vi "string parse mathematica assosiated array.vi"(7 "derivative":T2=enum."parse string", 10 "Map IN":map{T1, dbl}(c390), 11 "String in":string="74 -> <|\"m1\" -> 0.144686311901723`, \"m2\" -> 0.01872411095198769`, \n  \"m3\" -> 0.00012732395447351627`, \"T\" -> 0.249000, \n  \"\\[Zeta]\" -> 0.077915, \"\\[Tau]1\" -> 0.054530, \"\\[Tau]S\" -> 0.034022,\n   \"\\[Tau]N\" -> 0.048248, \"\\[Tau]C\" -> 0.002031, \n  \"\\[Kappa]0\" -> 0.000000001550, \"mm1\" -> 0.016334, \"mm2\" -> 0.128767,\n   \"mm3\" -> 0.000140|>,\n\n\n") -> (2 "Map OUT":map{T1, dbl}(c390), 3 "String OUT":string)   [LabVIEW 2020]
uses:
  3-lorentzian-parameters.ctl
  mathematica string map action.ctl
  3-lorentzian-heat-response action.ctl
  <vilib>/regexp/Match Regular Expression.xnode
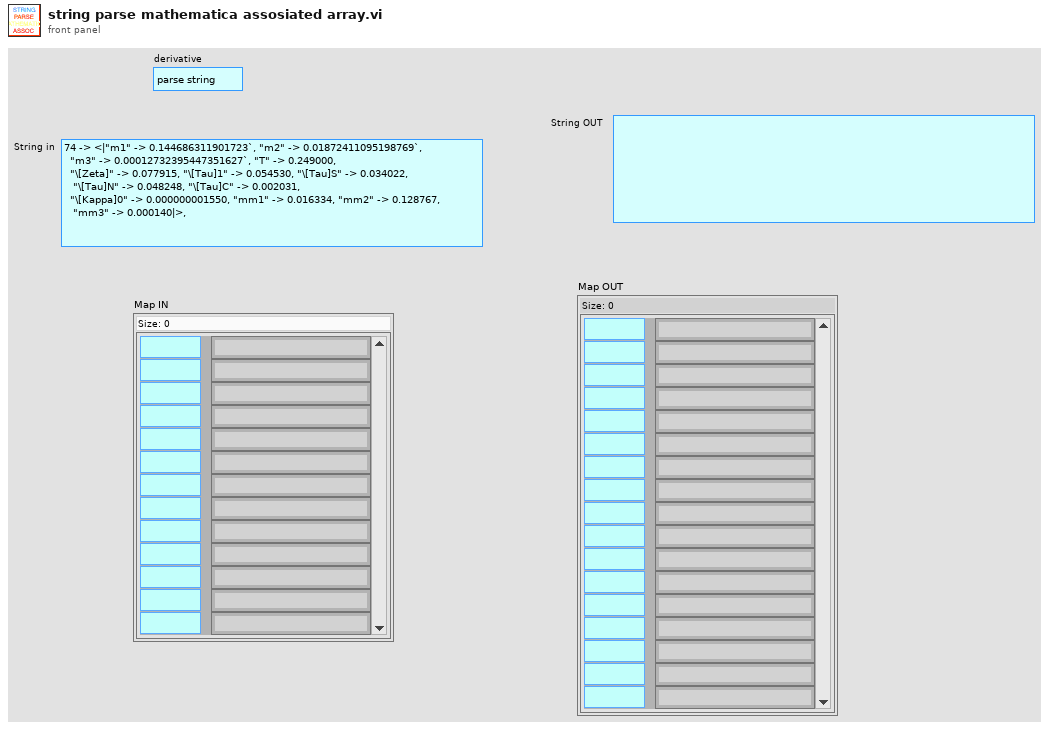
[diagram p1: front panel]
types:
  T1 = typedef "3-lorentzian-parameters.ctl" = enum16{"ζ", "τ1", "τS", "τN", "τC", "κ0", "m1", "m2", "m3", "T (K)", "B (T)", "θ (deg)"}
  T2 = typedef "mathematica string map action.ctl" = enum16{"create string", "calc m1m2m3", "parse string"}
  T3 = typedef "3-lorentzian-heat-response action.ctl" = enum16{"calc R", "create string", "calc m1m2m3", "dζ", "dT1", "dτS", "dτN", "dτC", "d-all", "dκ0", "T(K)", "m1", "m2", "m3", "parse string", "θ (deg)", "B (T)", "onlygrads"}
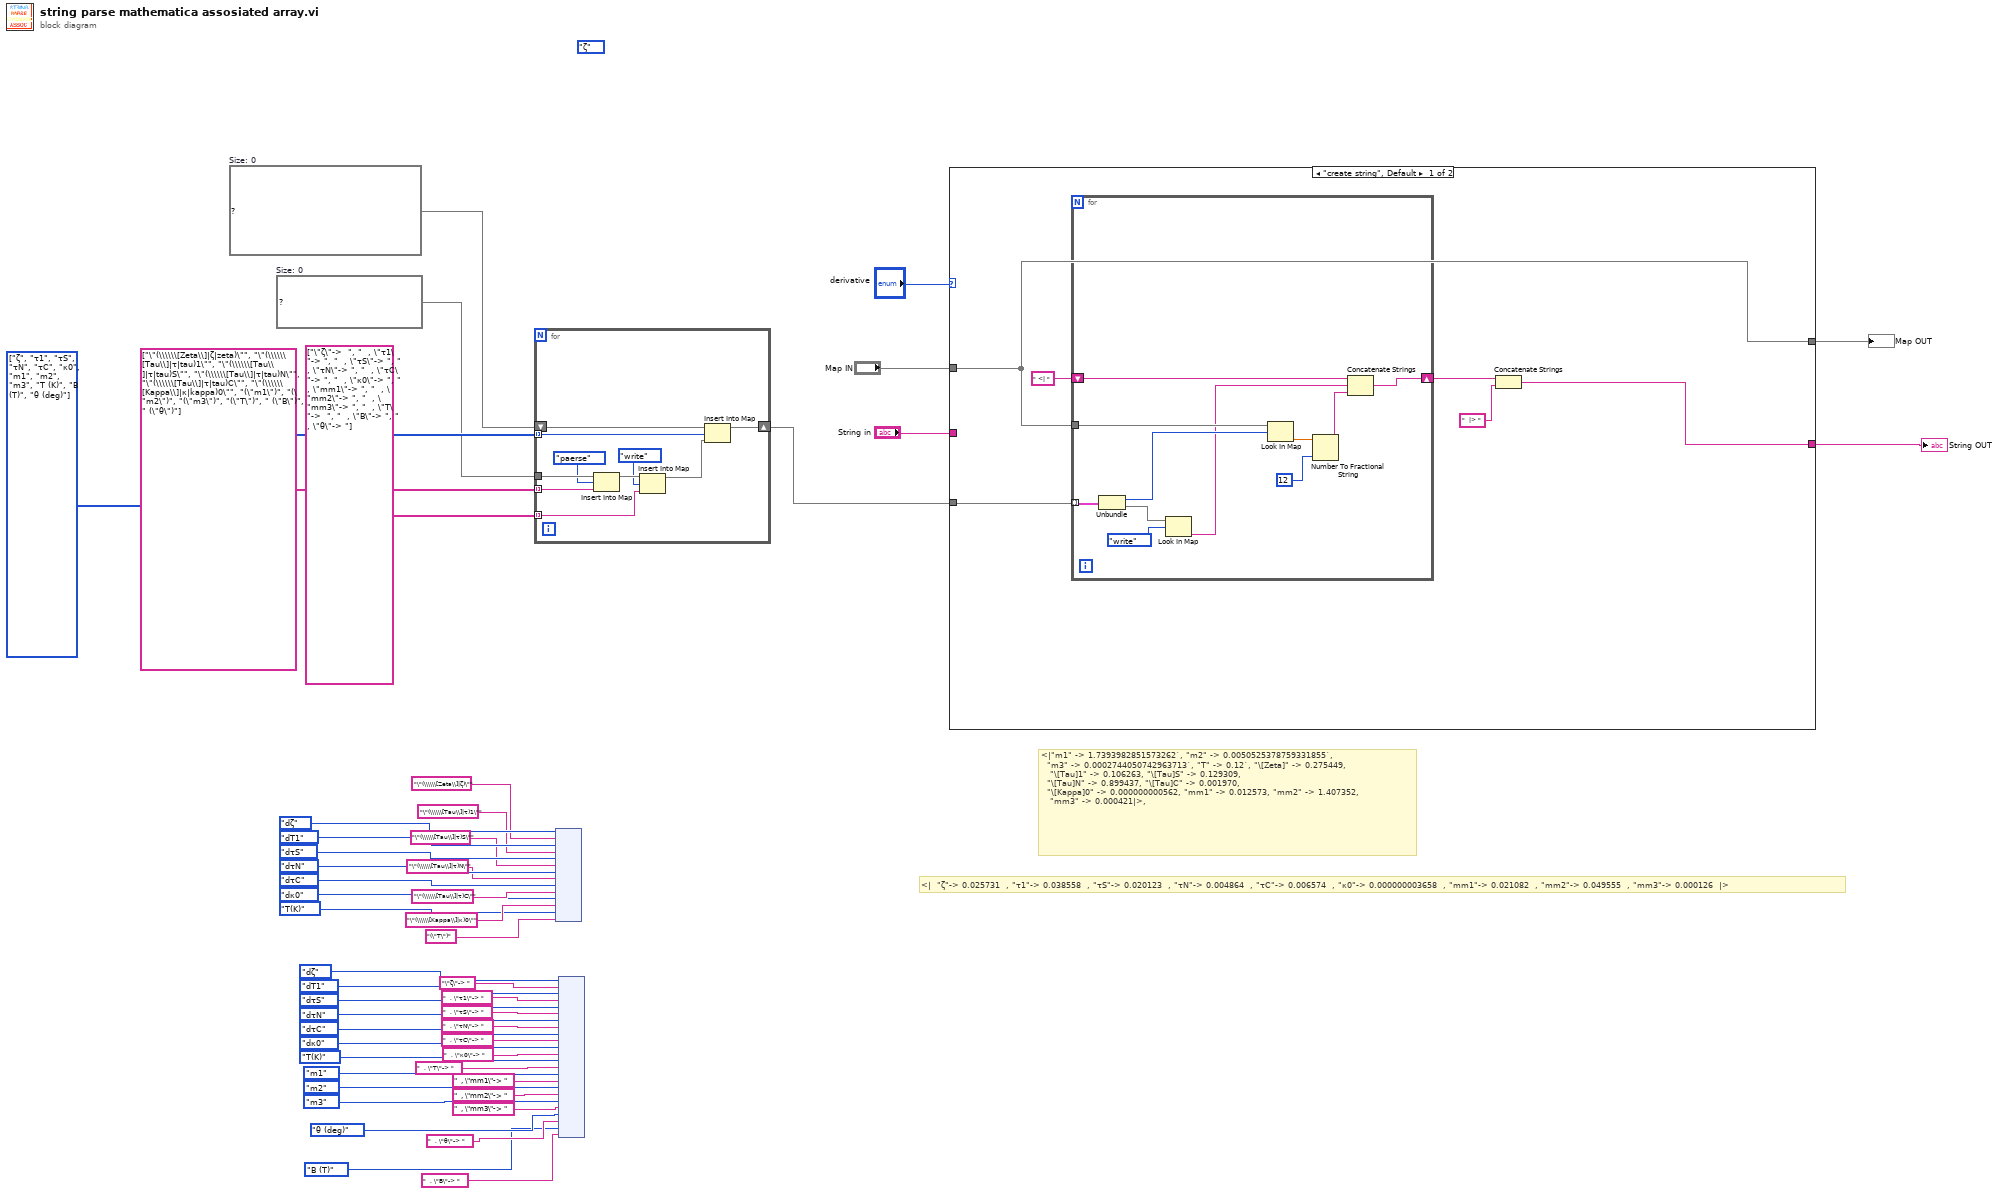
[diagram p0: block diagram]
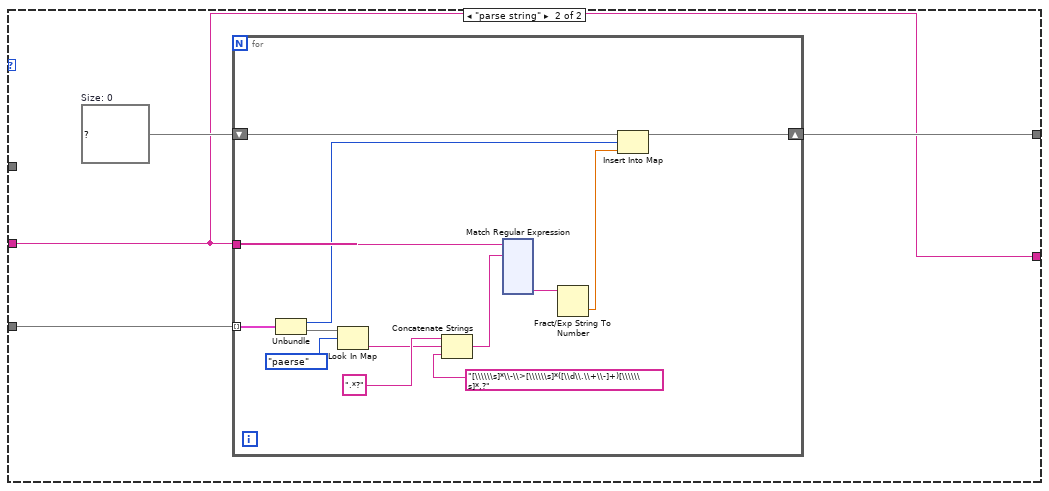
[diagram p2: hidden frame]
diagram:
  (unwired) 3-lorentzian-parameters."ζ" ("what")
  w5 = map{enum16{"paerse", "write"}, string} {}  # Size: 0
  w6 = map{T1, map{enum16{"paerse", "write"}, string}} {}  # Size: 0
  w7 = T1[] [enum."ζ", enum."τ1", enum."τS", enum."τN", enum."τC", enum."κ0", enum."m1", enum."m2", enum."m3", enum."T (K)", enum."B (T)", enum."θ (deg)"] items=["ζ", "τ1", "τS", "τN", "τC", "κ0", "m1", "m2", "m3", "T (K)", "B (T)", "θ (deg)"]
  # "<|\"m1\" -> 1.7393982851573262`, \"m2\" -> 0.0050525378759331855`, \n  \"m3\" -> 0.0002744050742963713`, \"T\" -> 0.12`, \"\\[Zeta]\" -> 0.275449,\n   \"\\[Tau]1\" -> 0.106263, \"\\[Tau]S\" -> 0.129309, \n  \"\\[Tau]N\" -> 0.899437, \"\\[Tau]C\" -> 0.001970, \n  \"\\[Kappa]0\" -> 0.000000000562, \"mm1\" -> 0.012573, \"mm2\" -> 1.407352,\n   \"mm3\" -> 0.000421|>,"
  # "<|  \"ζ\"-> 0.025731  , \"τ1\"-> 0.038558  , \"τS\"-> 0.020123  , \"τN\"-> 0.004864  , \"τC\"-> 0.006574  , \"κ0\"-> 0.000000003658  , \"mm1\"-> 0.021082  , \"mm2\"-> 0.049555  , \"mm3\"-> 0.000126  |>"
  n1 = for {
    tunnel: w7 -> [w57] mode=indexing
    shift-right: [w58] -> w2
    shift-left: w6 -> [w59]
    tunnel: w5 -> [w56]
    tunnel: string[] ["\"(\\\\\\[Zeta\\]|ζ|zeta)\"", "\"(\\\\\\[Tau\\]|τ|tau)1\"", "\"(\\\\\\[Tau\\]|τ|tau)S\"", "\"(\\\\\\[Tau\\]|τ|tau)N\"", "\"(\\\\\\[Tau\\]|τ|tau)C\"", "\"(\\\\\\[Kappa\\]|κ|kappa)0\"", "(\"m1\")", "(\"m2\")", "(\"m3\")", "(\"T\")", " (\"B\")", " (\"θ\")"] -> [w51] mode=indexing
    tunnel: string[] ["\"ζ\"->  ", "  , \"τ1\"-> ", "  , \"τS\"-> ", "  , \"τN\"-> ", "  , \"τC\"-> ", "  , \"κ0\"-> ", "  , \"mm1\"-> ", "  , \"mm2\"-> ", "  , \"mm3\"-> ", "  , \"T\"->  ", "  , \"B\"-> ", "  , \"θ\"-> "] -> [w50] mode=indexing
    n2 = Insert Into Map(map in=w56, key=enum16{"paerse", "write"}."paerse", value=w51) -> (map out=w55:map{enum16{"paerse", "write"}, string})  [unwired: 2 out]
    n3 = Insert Into Map(map in=w55, key=enum16{"paerse", "write"}."write", value=w50) -> (map out=w54:map{enum16{"paerse", "write"}, string})  [unwired: 2 out]
    n4 = Insert Into Map(map in=w59, key=w57, value=w54) -> (map out=w58:map{T1, map{enum16{"paerse", "write"}, string}})  [unwired: 2 out]
  }
  n5 = node(3-lorentzian-heat-response_action."dζ" ("derivative"), "\"(\\\\\\[Zeta\\]|ζ)\"" ("format string"), 3-lorentzian-heat-response_action."dT1" ("derivative"), "\"(\\\\\\[Tau\\]|τ)1\"" ("format string"), 3-lorentzian-heat-response_action."dτS" ("derivative"), "\"(\\\\\\[Tau\\]|τ)S\"" ("format string"), 3-lorentzian-heat-response_action."dτN" ("derivative"), "\"(\\\\\\[Tau\\]|τ)N\"" ("format string"), 3-lorentzian-heat-response_action."dτC" ("derivative"), "\"(\\\\\\[Tau\\]|τ)C\"" ("format string"), 3-lorentzian-heat-response_action."dκ0" ("derivative"), "\"(\\\\\\[Kappa\\]|κ)0\"" ("format string"), 3-lorentzian-heat-response_action."T(K)" ("derivative"), "(\"T\")" ("format string")) -> ()  [unwired: 1 out]
  n6 = node(3-lorentzian-heat-response_action."dζ" ("derivative"), "\"ζ\"-> ", 3-lorentzian-heat-response_action."dT1" ("derivative"), "  , \"τ1\"-> ", 3-lorentzian-heat-response_action."dτS" ("derivative"), "  , \"τS\"-> ", 3-lorentzian-heat-response_action."dτN" ("derivative"), "  , \"τN\"-> ", 3-lorentzian-heat-response_action."dτC" ("derivative"), "  , \"τC\"-> ", 3-lorentzian-heat-response_action."dκ0" ("derivative"), "  , \"κ0\"-> ", 3-lorentzian-heat-response_action."T(K)" ("derivative"), "  , \"T\"-> ", 3-lorentzian-heat-response_action."m1" ("derivative"), "  , \"mm1\"-> ", 3-lorentzian-heat-response_action."m2" ("derivative"), "  , \"mm2\"-> ", 3-lorentzian-heat-response_action."m3" ("derivative"), "  , \"mm3\"-> ", 3-lorentzian-heat-response_action."θ (deg)" ("derivative"), "  , \"θ\"-> ", 3-lorentzian-heat-response_action."B (T)" ("derivative"), "  , \"B\"-> ") -> ()  [unwired: 1 out]
  n7 = case shown="\"create string\", Default" "derivative" {
    tunnel: "String in" -> [_ w78]
    tunnel: [w61 w79] -> w1
    tunnel: [w62 w78] -> w47
    tunnel: w2 -> [w60 w77]
    tunnel: "Map IN" -> [w61 _]
    frame "create string", Default {
      n8 = for {
        shift-right: [w76] -> w64
        shift-left: " <| " -> [w72]
        tunnel: w60 -> [w69] mode=indexing
        tunnel: w61 -> [w75]
        n9 = Unbundle(w69) -> ("what"=w74:T1, w68:map{enum16{"paerse", "write"}, string})
        n10 = Look In Map(map=w68, key=enum16{"paerse", "write"}."write") -> (value=w66:string)  [unwired: 1 in, 1 out]
        n11 = Look In Map(map=w75, key=w74) -> (value=w73:dbl)  [unwired: 1 in, 1 out]
        n12 = Number To Fractional String(number=w73, precision (6)=i16 12) -> (F-format string=w71:string)  [unwired: 2 in]
        n13 = Concatenate Strings(w72, w66, w71) -> (w76:string)
      }
      n14 = Concatenate Strings(w64, "  |> ") -> (w62:string)
    }
    frame "parse string" {
      w80 = map{T1, dbl} {}  # Size: 0
      n15 = for {
        tunnel: w77 -> [w87] mode=indexing
        tunnel: w78 -> [w89]
        shift-right: [w84] -> w79
        shift-left: w80 -> [w88]
        n16 = Unbundle(w87) -> ("what"=w86:T1, w83:map{enum16{"paerse", "write"}, string})
        n17 = Look In Map(map=w83, key=enum16{"paerse", "write"}."paerse") -> (value=w81:string)  [unwired: 1 in, 1 out]
        n18 = Concatenate Strings(".*?" ("format string"), w81, "[\\\\\\s]*\\-\\>[\\\\\\s]*([\\d\\.\\+\\-]+)[\\\\\\s]*,?" ("format string")) -> (w90:string)
        n19 = xnode "Match Regular Expression"("input string"=w89, "regular expression"=w90) -> ("submatch 2"=w93:string)  [unwired: 4 in, 6 out]
        n20 = Fract/Exp String To Number(string=w93) -> (number=w85:dbl)  [unwired: 3 in, 1 out]
        n21 = Insert Into Map(map in=w88, key=w86, value=w85) -> (map out=w84:map{T1, dbl})  [unwired: 2 out]
      }
    }
  }
  "Map OUT" <- w1
  "String OUT" <- w47
